vi "SLSC Get Module Name from IP Address.vi"(5 "Password":string, 6 "connect timeout":dbl=50.0, 7 "Username":string="admin", 8 "Error In":errorcluster, 10 "Slot #":u32=4, 11 "Chassis IP Address":string="192.168.0.14") -> (0 "Error Out":errorcluster, 1 "SLSC Chassis Name":string, 3 "SLSC Module Name":string)   [LabVIEW 2015, in "SLSC EDS Engine.lvlib"]
uses:
  SLSC EDS Engine.lvlib
  <vilib>/nisyscfg/Close (System).vi
  <vilib>/SLSC/Initialize Session with Devices.vi
  <vilib>/SLSC/Initialize Session without Resources.vi
  <vilib>/SLSC/Close Session.vi
  <vilib>/SLSC/SLSC.lvlib
  <resource>/objmgr/slsc.rc
  <vilib>/nisyscfg/nisyscfg.lvlib
  <resource>/objmgr/nisysapi.rc
  SLSC EDS API/SLSC EDS API.lvlib
panel:
  out "chassis debug":string
  out "session out debug":string
  out "Dev.SlotNum":u32
  out "Module Found?":bool
  out "Host Name":string
  out "Dev.Modules":string[](array[string])
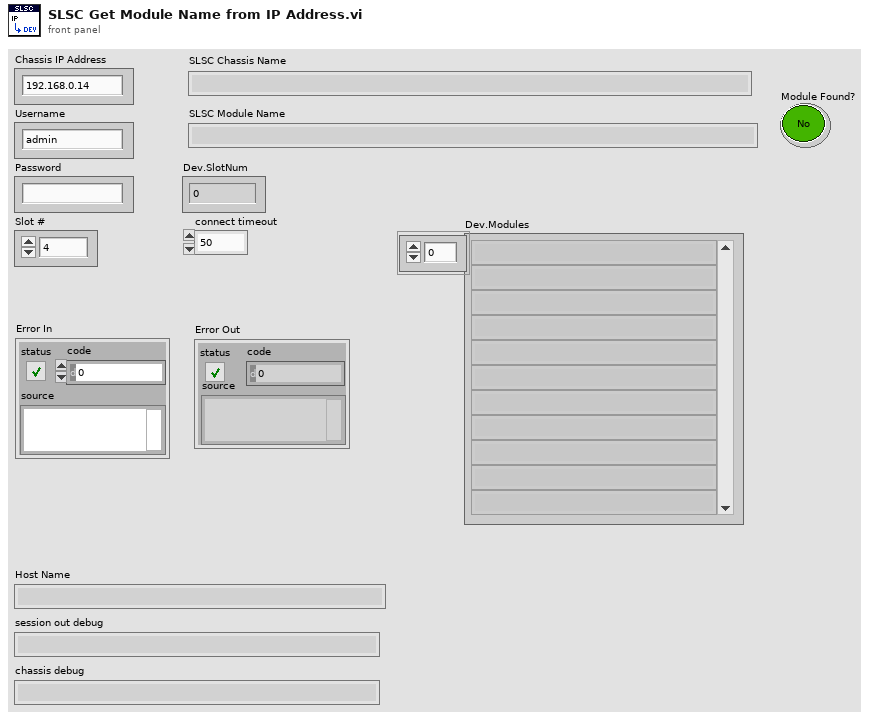
[diagram p1: front panel]
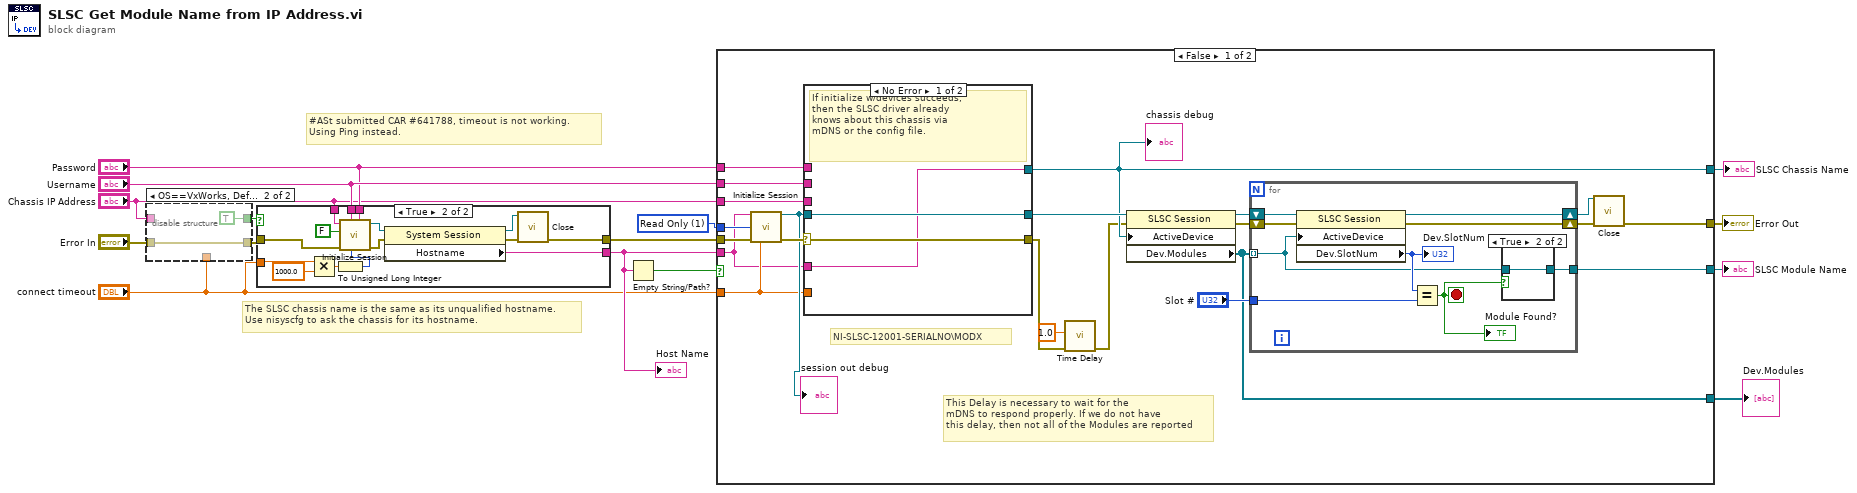
[diagram p0: block diagram]
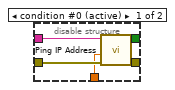
[diagram p2: hidden frame]
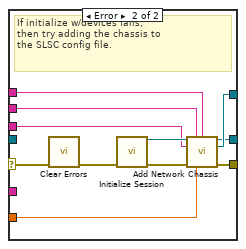
[diagram p4: hidden frame]
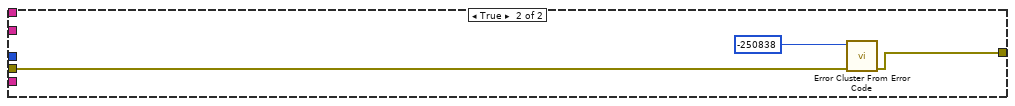
[diagram p6: hidden frame]
diagram:
  w13 = 1 items=["None"=0, "Read Only"=1, "Read/Write"=3] ("reservation access (Read/Write)")
  # "#ASt submitted CAR #641788, timeout is not working.\nUsing Ping instead."
  # "The SLSC chassis name is the same as its unqualified hostname.\nUse nisyscfg to ask the chassis for its hostname."
  n1 = disable-structure shown="OS==VxWorks, Default" {
    disable-tunnel: "Chassis IP Address" -> [w20 _]
    disable-tunnel: [w19 TRUE ("response?")] -> w5
    disable-tunnel: "Error In" -> [w18 w22]
    disable-tunnel: [w17 w22] -> w3
    disable-tunnel: "connect timeout" -> [w16 _]
    frame condition #0 (active) {
      n2 = call "Ping IP Address.vi"("error in"=w18, "timeout (500 ms)"=w16, "host"=w20) -> ("error out"=w17:errorcluster, "response?"=w19:bool)  [unwired: 6 in, 1 out]
    }
    frame condition #1 {
    }
  }
  n3 = case shown="True" w5 {
    tunnel: [w23 w34] -> w14
    tunnel: w3 -> [w23 w30]
    tunnel: "Username" -> [_ w29]
    tunnel: "Password" -> [_ w28]
    tunnel: "connect timeout" -> [_ w27]
    tunnel: [_ w25] -> w7
    tunnel: "Chassis IP Address" -> [_ w24]
    frame False {
    }
    frame True {
      n4 = Multiply(x=w27, y=1000.0) -> (x*y=w32:dbl)
      n5 = To Unsigned Long Integer(number=w32) -> (unsigned 32bit integer=w31:u32)
      n6 = call <vilib>:"Initialize Session.vi"("Password"=w28, "Connect Timeout (4000 ms)"=w31, "User Name"=w29, "error in (no error)"=w30, "Force Property Refresh (T)"=FALSE, "Target (localhost)"=w24) -> ("error out"=w37:errorcluster, "Session out"=w38:refnum<k21>)  [unwired: 4 in]
      n7 = property class="System Session"(reference=w38, error in=w37) -> (reference out=w35:refnum<k21>, error out=w36:errorcluster, "Hostname"=w25:string)
      n8 = call-poly <vilib>:"Close.vi"("error in (no error)"=w36, "Session in"=w35) -> ("error out"=w34:errorcluster)  [unwired: 9 in]
    }
  }
  "Host Name" <- w7
  n9 = Empty String/Path?(string/path=w7) -> (empty?=w8:bool)
  n10 = case shown="False" w8 {
    tunnel: [w43 w87] -> w15
    tunnel: w14 -> [w56 w85]
    tunnel: w13 -> [w55 _]
    tunnel: "Chassis IP Address" -> [w52 _]
    tunnel: "Username" -> [w51 _]
    tunnel: "Password" -> [w50 _]
    tunnel: [w48 _] -> w10
    tunnel: "connect timeout" -> [w46 _]
    tunnel: [w45 _] -> w9
    tunnel: w7 -> [w44 _]
    tunnel: [w39 _] -> w1
    frame False {
      # "This Delay is necessary to wait for the \nmDNS to respond properly. If we do not have\nthis delay, then not all of the Modules are reported"
      # "NI-SLSC-12001-SERIALNO\\MODX"
      n11 = call-poly <vilib>:"Initialize Session.vi"("devices"=w44, "reservation access (Read/Write)"=w55, "error in (no error)"=w56, "connect timeout (60 sec)"=w46) -> ("session out"=w53:refnum<k21>, "error out"=w54:errorcluster)  [unwired: 10 in]
      "session out debug" <- w53
      n12 = case shown="No Error" w54 {
        selector: w54 -> [w63 w74]
        tunnel: [w63 w66] -> w42
        tunnel: [w62 w67] -> w49
        tunnel: w53 -> [w62 _]
        tunnel: w52 -> [_ w72]
        tunnel: w51 -> [_ w70]
        tunnel: w50 -> [_ w69]
        tunnel: [w61 w68] -> w48
        tunnel: w44 -> [w61 _]
        tunnel: w46 -> [_ w64]
        frame No Error {
          # "If initialize w/devices succeeds,\nthen the SLSC driver already\nknows about this chassis via\nmDNS or the config file."
        }
        frame Error {
          # "If initialize w/devices fails,\nthen try adding the chassis to\nthe SLSC config file."
          n13 = call <vilib>:"Clear Errors.vi"("error in (no error)"=w74) -> ("error out"=w65:errorcluster)  [unwired: 5 in, 1 out]
          n14 = call-poly <vilib>:"Initialize Session.vi"("error in (no error)"=w65) -> ("session out"=w73:refnum<k21>, "error out"=w71:errorcluster)  [unwired: 13 in]
          n15 = call <vilib>:"Add Network Chassis.vi"("session in"=w73, "username"=w70, "password"=w69, "chassis IP address/hostname"=w72, "error in (no error)"=w71, "connect timeout (60 sec)"=w64) -> ("session out"=w67:refnum<k21>, "chassis out"=w68:refnum<k21>, "error out"=w66:errorcluster)  [unwired: 7 in]
        }
      }
      "chassis debug" <- w48
      n16 = call "Time Delay"("error in (no error)"=w42, "Delay Time (s)"=1.0) -> ("error out"=w41:errorcluster)  [unwired: 9 in]
      n17 = property class="SLSC Session"(reference=w49, error in=w41, "ActiveDevice"=w48) -> (reference out=w59:refnum<k21>, error out=w58:errorcluster, "Dev.Modules"=w39:refnum<k21>[])
      n18 = for {
        tunnel: w39 -> [w77] mode=indexing
        tunnel: "Slot #" -> [w83]
        tunnel: [w76] -> w45
        shift-right: [w79] -> w47
        shift-left: w58 -> [w80]
        shift-right: [w78] -> w57
        shift-left: w59 -> [w82]
        stop <- w75 stop-if-true
        n19 = property class="SLSC Session"(reference=w82, error in=w80, "ActiveDevice"=w77) -> (reference out=w78:refnum<k21>, error out=w79:errorcluster, "Dev.SlotNum"=w81:u32)
        "Dev.SlotNum" <- w81
        n20 = Equal?(x=w81, y=w83) -> (x = y?=w75:bool)
        "Module Found?" <- w75
        n21 = case shown="True" w75 {
          tunnel: w77 -> [_ w84]
          tunnel: [_ w84] -> w76
          frame False {
          }
          frame True {
          }
        }
      }
      n22 = call-poly <vilib>:"Close.vi"("session in"=w57, "error in (no error)"=w47) -> ("error out"=w43:errorcluster)  [unwired: 13 in]
    }
    frame True {
      n23 = call <vilib>:"Error Cluster From Error Code.vi"("error in (no error)"=w85, "error code (0)"=-250838 ("code")) -> ("error out"=w87:errorcluster)  [unwired: 7 in]
    }
  }
  "SLSC Chassis Name" <- w10
  "Error Out" <- w15
  "SLSC Module Name" <- w9
  "Dev.Modules" <- w1
